vi "Keithley2400series_MUX_2t.vi"() -> ()   [LabVIEW 2014]
panel:
  out "VISA resource name out":refnum<visa-resource-name>
  out "error out":errorcluster
  in  "Numeric":u8 max=15
  in  "VISA resource name 2":refnum<visa-resource-name>
  in  "Serial Configuration":T1={"Baud Rate"=9600, "Parity"=0, "Data Bits"=8, "Stop Bits"=10, "Flow Control"=0} {"Flow Control" items=["None", "XON/XOFF", "RTS/CTS", "XON/XOFF & RTS/CTS", "DTR/DSR", "XON/XOFF & DTR/DSR"]; "Stop Bits" items=["1.0"=10, "1.5"=15, "2.0"=20]; "Data Bits" items=["7"=7, "8"=8]; "Parity" items=["None", "Odd", "Even", "Mark", "Space"]; "Baud Rate" items=["300"=300, "600"=600, "1200"=1200, "2400"=2400, "4800"=4800, "9600"=9600, "19200"=19200]}
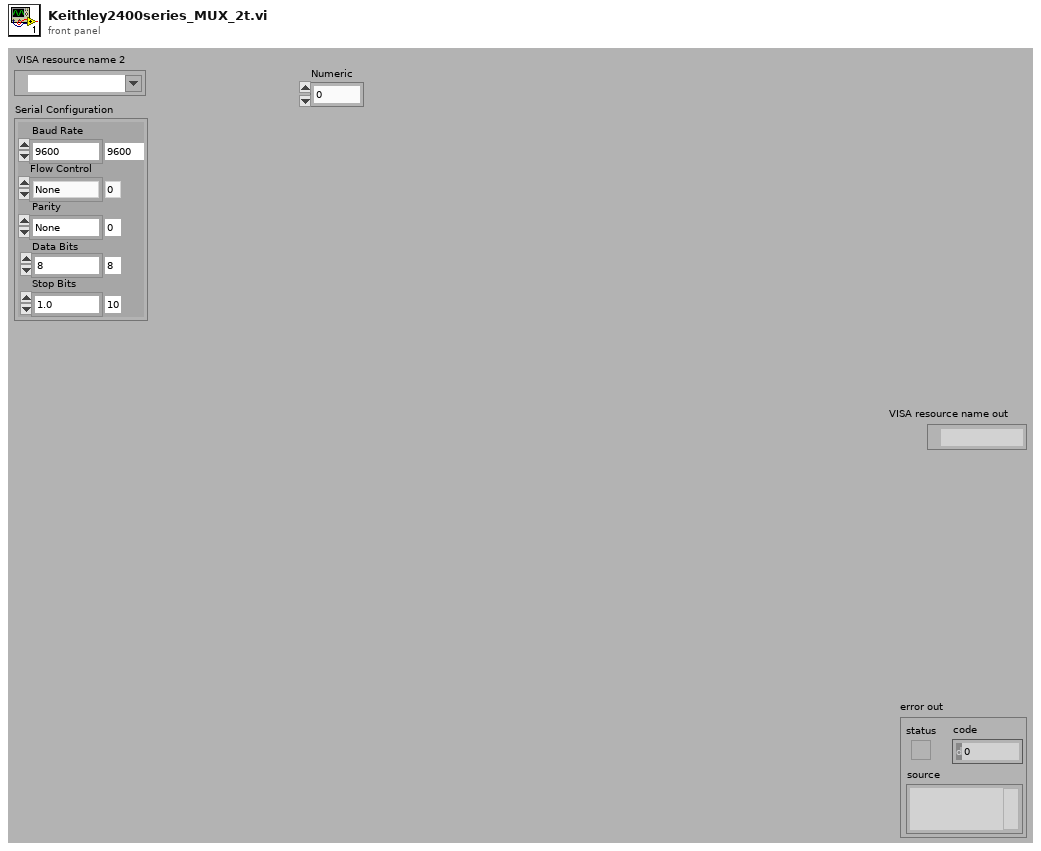
[diagram p1: front panel]
types:
  T1 = cluster{"Baud Rate":u32, "Parity":u16, "Data Bits":u16, "Stop Bits":u16, "Flow Control":u16}
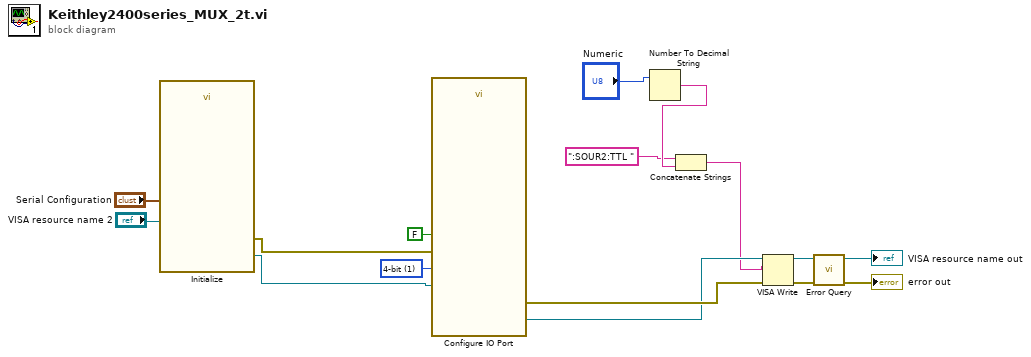
[diagram p0: block diagram]
diagram:
  w12 = u16 1 items=["3-bit", "4-bit"] ("Operating Mode (0: 3-bit)")
  n1 = call "Initialize.vi"("Serial Configuration"="Serial Configuration", "VISA resource name"="VISA resource name 2") -> ("error out"=w14:errorcluster, "VISA resource name out"=w13:refnum<visa-resource-name>)  [unwired: 8 in]
  n2 = call "Configure IO Port.vi"("error in (no error)"=w14, "Enable Auto Clear (T:Enable)"=FALSE, "Operating Mode (0: 3-bit)"=w12, "VISA resource name"=w13) -> ("error out"=w3:errorcluster, "VISA resource name out"=w2:refnum<visa-resource-name>)  [unwired: 6 in]
  n3 = Number To Decimal String(number="Numeric") -> (decimal integer string=w5:string)  [unwired: 1 in]
  n4 = Concatenate Strings(":SOUR2:TTL " ("string"), w5) -> (w1:string)
  n5 = VISA Write(VISA resource name=w2, write buffer=w1, error in (no error)=w3) -> (VISA resource name out=w8:refnum<visa-resource-name>, error out=w7:errorcluster)  [unwired: 1 out]
  n6 = call "Error Query.vi"("error in (no error)"=w7, "VISA resource name"=w8) -> ("error out"=→"error out":errorcluster, "VISA resource name out"=→"VISA resource name out":refnum<visa-resource-name>)  [unwired: 6 in, 2 out]
